vi "add_installer_location.vi"   [LabVIEW 2015, in "lv-post-installer.lvlib"]
uses:
  lv-post-installer.lvlib
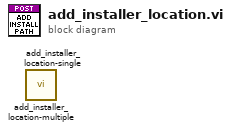
[diagram p0: block diagram]
diagram:
  n1 = call "add_installer_location-multiple.vi"() -> ()  [unwired: 11 in, 1 out]
  n2 = call "add_installer_location-single.vi"() -> ()  [unwired: 11 in, 1 out]
